vi "Init.vi"(8 "error in (no error)":errorcluster, 11 "AverageCollector1D in":refnum<class "AverageCollector1D.lvclass">) -> (0 "error out":errorcluster, 3 "AverageCollector1D out":refnum<class "AverageCollector1D.lvclass">)   [LabVIEW 2014, in "AverageCollector1D.lvclass"]
uses:
  AverageCollector1D.lvclass
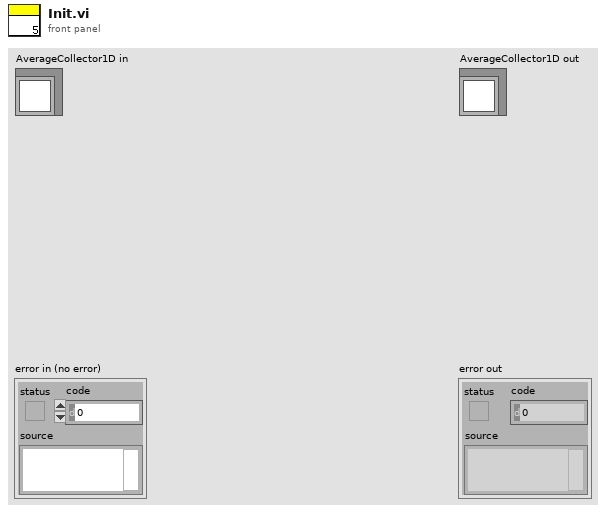
[diagram p1: front panel]
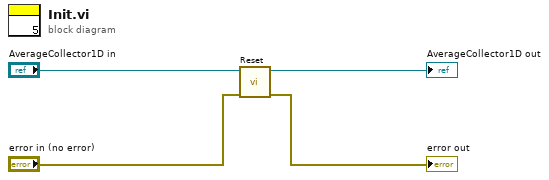
[diagram p0: block diagram]
diagram:
  n1 = call-dynamic "Reset.vi"("error in (no error)"="error in (no error)", "AbstractCollector1D in"="AverageCollector1D in") -> ("error out"=→"error out":errorcluster, "AbstractCollector1D out"=→"AverageCollector1D out":refnum<class "AverageCollector1D.lvclass">)  [unwired: 8 in]
